vi "Load Programs.vi"(0 "Program List in":refnum<class "Program List From File.lvclass">, 5 "error in (no error)":errorcluster, 8 "Application.lvclass":refnum<class "Application.lvclass">) -> (14 "Program List out":refnum<class "Program List From File.lvclass">, 15 "Programs":string[](array[string]), 19 "error out":errorcluster)   [LabVIEW 2019, in "Program List From File.lvclass"]
uses:
  Program List From File.lvclass
  Application.lvclass
  <vilib>/Utility/config.llb/NI_LVConfig.lvlib
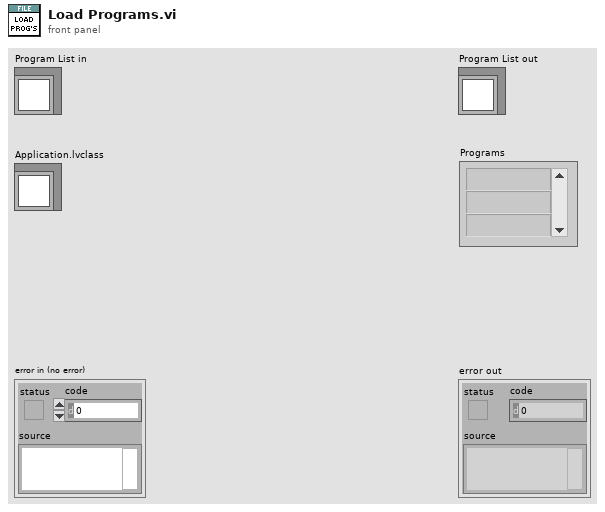
[diagram p1: front panel]
types:
  T1 = typedef "NI_LVConfig.lvlib/Config Data RefNum.ctl" = refnum<k1>
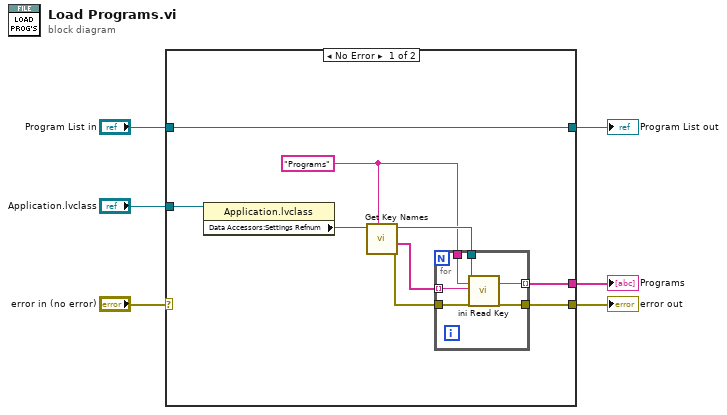
[diagram p0: block diagram]
diagram:
  n1 = case shown="No Error" "error in (no error)" {
    selector: "error in (no error)" -> [_ w23]
    tunnel: [w7 w23] -> w1
    tunnel: [w15 w22] -> w3
    tunnel: "Program List in" -> [w15 w22]
    tunnel: "Application.lvclass" -> [w9 _]
    tunnel: [w8 _] -> w2
    frame No Error {
      w10 = "Programs" ("section")
      n2 = property class="Application.lvclass"(reference=w9) -> ("Data Accessors:Settings Refnum"=w14:T1)  [unwired: 1 in, 2 out]
      n3 = call <vilib>:"Get Key Names.vi"("section"=w10, "refnum"=w14) -> ("error out"=w12:errorcluster, "key names"=w11:string[], "refnum out"=w13:T1)  [unwired: 6 in, 1 out]
      n4 = for {
        tunnel: w13 -> [w21]
        tunnel: w12 -> [w20]
        tunnel: w11 -> [w19] mode=indexing
        tunnel: w10 -> [w18]
        tunnel: [w17] -> w7
        tunnel: [w16] -> w8 mode=indexing
        n5 = call "ini Read Key.vi"("Refnum in"=w21, "Section"=w18, "Key"=w19, "Error In"=w20) -> ("value"=w16:string, "error out"=w17:errorcluster)  [unwired: 13 in, 1 out]
      }
    }
    frame Error {
    }
  }
  "error out" <- w1
  "Program List out" <- w3
  "Programs" <- w2
